vi "4.7.vi"() -> ()   [LabVIEW 2017]
panel:
  out "随机的数":i16
  out "循环次数":dbl
  in  "猜测的数":i16
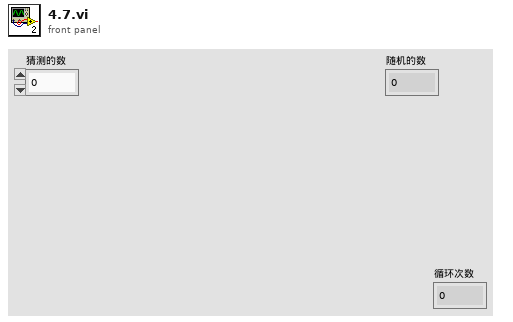
[diagram p1: front panel]
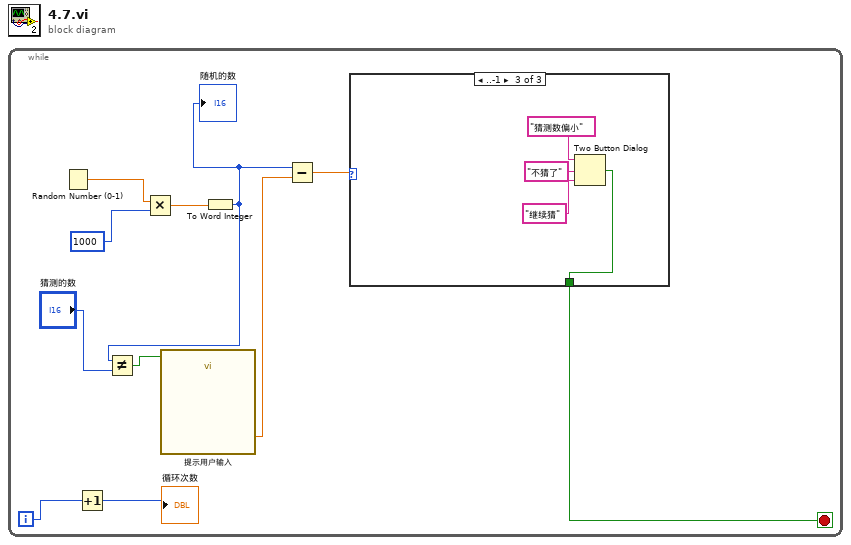
[diagram p0: block diagram]
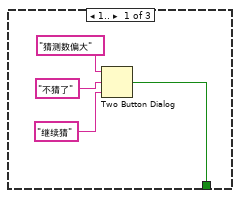
[diagram p2: hidden frame]
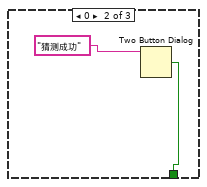
[diagram p3: hidden frame]
diagram:
  n1 = while {
    i -> [w9]
    stop <- w2 stop-if-true
    n2 = Random Number (0-1)() -> (number: 0 to 1=w5:dbl)
    n3 = Increment(x=w9) -> (x+1=→"循环次数":i32)
    n4 = Multiply(x=w5, y=1000) -> (x*y=w10:dbl)
    n5 = To Word Integer(number=w10) -> (16bit integer=w1:i16)
    "随机的数" <- w1
    n6 = Not Equal?(x=w1, y="猜测的数") -> (x != y?=w6:bool)
    n7 = call "提示用户输入"("Enable"=w6) -> ("请在1—1000猜"=w3:dbl)  [unwired: 16 in, 2 out]
    n8 = Subtract(x=w1, y=w3) -> (x-y=w7:dbl)
    n9 = case shown="..-1" w7 {
      tunnel: [w12 w16 w18] -> w2
      frame 1.. {
        n10 = Two Button Dialog(message="猜测数偏大", 1:"继续猜", 2:"不猜了") -> (T button?=w12:bool)
      }
      frame 0 {
        n11 = Two Button Dialog(message="猜测成功") -> (T button?=w16:bool)  [unwired: 2 in]
      }
      frame ..-1 {
        n12 = Two Button Dialog(message="猜测数偏小", 1:"继续猜", 2:"不猜了") -> (T button?=w18:bool)
      }
    }
  }
